vi "Averaged Results.vi"(1 "Points to averages":i32) -> (0 "Averaged Result":dbl[][](array[numeric]))   [LabVIEW 2013]
uses:
  Lock-in Globals Multiple Inputs and Outputs.vi
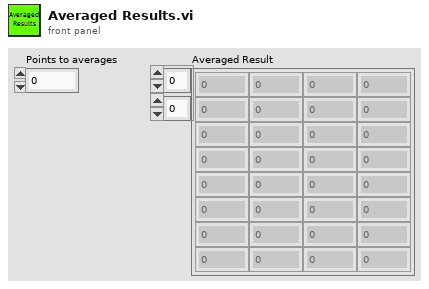
[diagram p1: front panel]
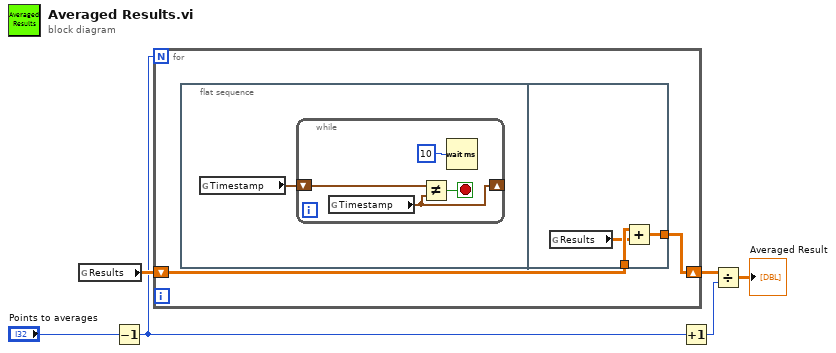
[diagram p0: block diagram]
diagram:
  n1 = global read "Lock-in Globals Multiple Inputs and Outputs.vi" "Results"() -> (w6:dbl[][])
  n2 = Decrement(x="Points to averages") -> (x-1=w3:i32)
  n3 = for {
    N: w3 -> [_]
    shift-right: [w7] -> w4
    shift-left: w6 -> [w8]
    n4 = flat-sequence {
      tunnel: w8 -> [w16]
      tunnel: [w14] -> w7
      frame #0 {
        n5 = global read "Lock-in Globals Multiple Inputs and Outputs.vi" "Timestamp"() -> (w9:timestamp)
        n6 = while {
          shift-right: [w10] -> _
          shift-left: w9 -> [w13]
          stop <- w11 stop-if-true
          n7 = global read "Lock-in Globals Multiple Inputs and Outputs.vi" "Timestamp"() -> (w10:timestamp)
          n8 = Not Equal?(x=w13, y=w10) -> (x != y?=w11:bool)
          n9 = Wait (ms)(milliseconds to wait=u32 10) -> ()  [unwired: 1 out]
        }
      }
      frame #1 {
        n10 = global read "Lock-in Globals Multiple Inputs and Outputs.vi" "Results"() -> (w15:dbl[][])
        n11 = Add(x=w16, y=w15) -> (x+y=w14:dbl[][])
      }
    }
  }
  n12 = Increment(x=w3) -> (x+1=w2:i32)
  n13 = Divide(x=w4, y=w2) -> (x/y=→"Averaged Result":dbl[][])
